vi "camera mjpeg.vi"(11 "CameraDevRef":T1) -> ()   [LabVIEW 2014]
uses:
  <vilib>/Rock Robotics/WPI/Camera/WPI_CameraDevRef.ctl
  <vilib>/Rock Robotics/WPI/Camera/WPI_CameraSettings Operations.ctl
  typedefs/vision/vision enable.ctl
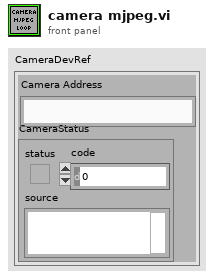
[diagram p1: front panel]
types:
  T1 = typedef "WPI_CameraDevRef.ctl" = cluster{"Camera Address":string, "CameraStatus":errorcluster}
  T2 = typedef "WPI_CameraSettings Operations.ctl" = enum16{"Udate FPS", "Update Compression", "Update Size", "Update White Balance", "Update Brightness", "Update Sharpness", "Update Exposure", "Update Exposure Value", "Update Color Level", "Update Exp Priority", "Update Color Enable", "Update JPG", "Update MJPG", "Read and Clear", "Read", "Init"}
  T3 = typedef "vision enable.ctl" = enum16{"Enable", "Disable", "Stop"}
  T4 = typedef "WPI_CameraSettings Control.ctl" = cluster{"FPS":i32, "Compression":i32, "Size":i32, "White Balance":i32, "Brightness":i32, "Sharpness":i32, "Exposure":i32, "Color Level":i32, "Exposure Priority":i32, "Color Enable":i32, "JPG Loop":i32, "MJPG Loop":i32, "Exposure Value":i32}
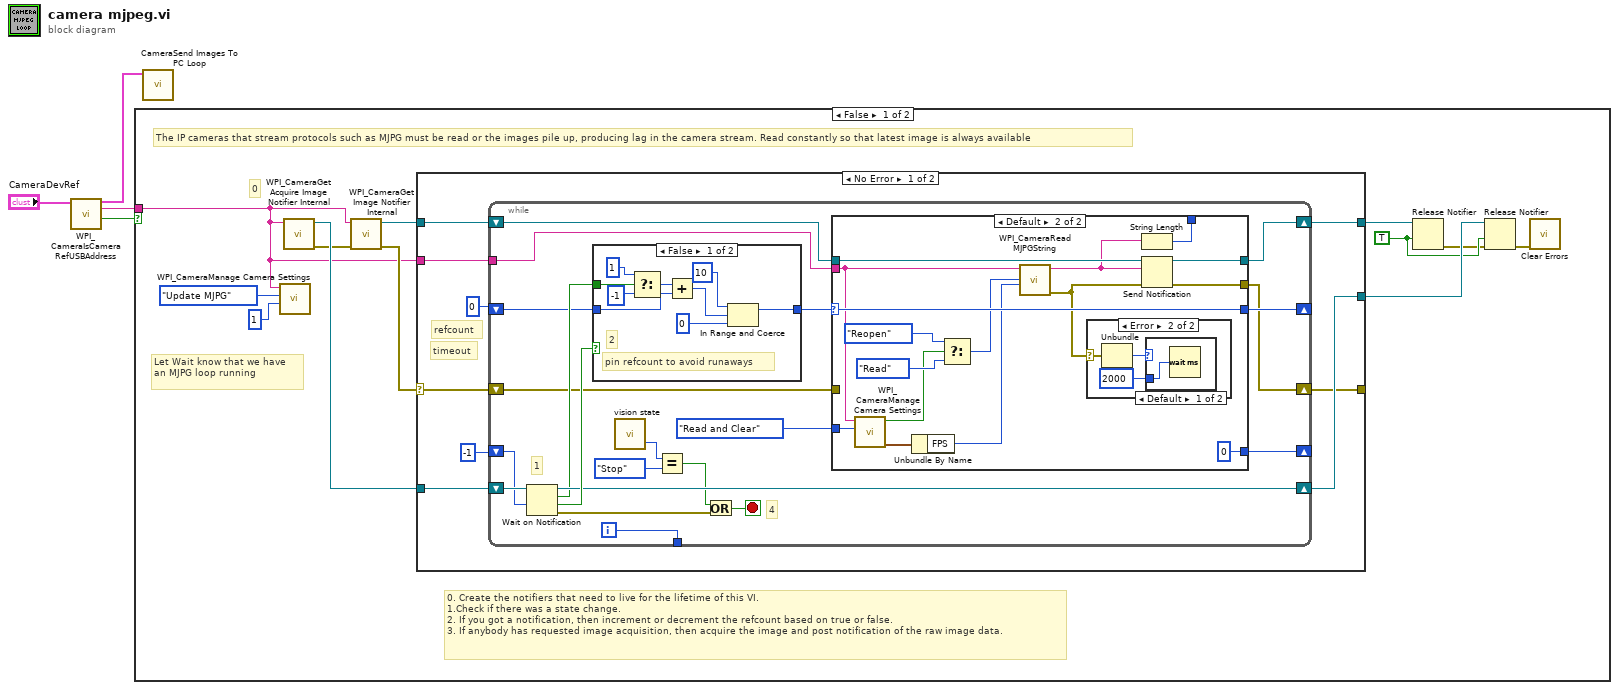
[diagram p0: block diagram]
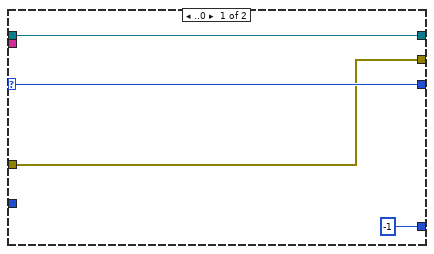
[diagram p2: hidden frame]
diagram:
  n1 = call <vilib>:"WPI_CameraIsCameraRefUSBAddress.vi"("CameraDevRef"="CameraDevRef") -> ("USB?"=w3:bool, "Camera Address Out"=w2:string, "CameraDevRef out"=w1:T1)  [unwired: 7 in, 1 out]
  n2 = case shown="False" w3 {
    tunnel: w2 -> [w6 _]
    frame False {
      w13 = TRUE ("force destroy? (F)")
      # "The IP cameras that stream protocols such as MJPG must be read or the images pile up, producing lag in the camera stream. Read constantly so that latest image is always available"
      # "0. Create the notifiers that need to live for the lifetime of this VI. \n1.Check if there was a state change.\n2. If you got a notification, then increment or decrement the refcount based on true or false.\n3. If anybody has requested image acquisition, then acquire the image and post notification of the raw image data."
      # "Let Wait know that we have\nan MJPG loop running"
      # "0"
      n3 = call <vilib>:"WPI_CameraManage Camera Settings.vi"("Value"=1, "Operation"=WPI_CameraSettings_Operations."Update MJPG", "Camera IP"=w6) -> ()  [unwired: 7 in, 2 out]
      n4 = call <vilib>:"WPI_CameraGet Acquire Image Notifier Internal.vi"("Camera Address"=w6) -> ("error out"=w10:errorcluster, "Acquire Image Notifier"=w11:refnum<notifier>)  [unwired: 1 in, 8 out]
      n5 = call <vilib>:"WPI_CameraGet Image Notifier Internal.vi"("error in (no error)"=w10, "Camera Address"=w6) -> ("error out"=w12:errorcluster, "Image Notifier"=w14:refnum<notifier>)  [unwired: 8 out]
      n6 = case shown="No Error" w12 {
        selector: w12 -> [w18 w83]
        tunnel: w6 -> [w25 _]
        tunnel: w11 -> [w24 w81]
        tunnel: w14 -> [w22 w82]
        tunnel: [w20 w82] -> w16
        tunnel: [w19 w81] -> w15
        tunnel: [w17 w83] -> _
        frame No Error {
          # "timeout"
          # "refcount"
          n7 = while {
            shift-right: [w44] -> w19
            shift-left: w24 -> [w46]
            tunnel: w25 -> [w41]
            shift-right: [w34] -> _
            shift-left: 0 -> [w42]
            shift-right: [w39] -> w20
            shift-left: w22 -> [w40]
            shift-right: [w37] -> _
            shift-left: -1 -> [w38]
            shift-right: [w33] -> w17
            shift-left: w18 -> [w36]
            tunnel: [w31] -> _
            i -> [w31]
            stop <- w28 stop-if-true
            # "4"
            # "1"
            n8 = Wait on Notification(notifier=w46, timeout in ms (-1)=w38) -> (notifier out=w44:refnum<notifier>, notification=w43:bool, timed out?=w45:bool, error out=w27:errorcluster)  [unwired: 1 in, 1 out]
            n9 = case shown="False" w45 {
              tunnel: w43 -> [w79 _]
              tunnel: w42 -> [w75 w80]
              tunnel: [w71 w80] -> w35
              frame False {
                # "pin refcount to avoid runaways"
                # "2"
                n10 = Select(t=1, s=w79, f=-1) -> (s? t:f=w76:i32)
                n11 = Add(x=w76, y=w75) -> (x+y=w72:i32)
                n12 = In Range and Coerce(upper limit=10, x=w72, lower limit=0) -> (coerced(x)=w71:i32)  [unwired: 1 out]
              }
              frame True {
              }
            }
            n13 = call "vision state.vi"() -> ("State Out"=w30:T3)  [unwired: 2 in, 1 out]
            n14 = Equal?(x=w30, y=vision_enable."Stop") -> (x = y?=w26:bool)
            n15 = Or(x=w26, y=w27) -> (x .or. y?=w28:bool)
            n16 = case shown="Default" w35 {
              selector: w35 -> [w49 w63]
              tunnel: w41 -> [_ w51]
              tunnel: w40 -> [w50 w66]
              tunnel: [w50 w65] -> w39
              tunnel: [-1 0] -> w37
              tunnel: w36 -> [w47 _]
              tunnel: [w49 w63] -> w34
              tunnel: [w47 w62] -> w33
              tunnel: [_ w56] -> _
              tunnel: WPI_CameraSettings_Operations."Read and Clear" ("Operation") -> [_ w52]
              frame ..0 {
              }
              frame Default {
                n17 = call <vilib>:"WPI_CameraManage Camera Settings.vi"("Operation"=w52, "Camera IP"=w51) -> ("Values"=w54:T4, "Changed"=w55:bool)  [unwired: 8 in]
                n18 = Unbundle By Name(w54) -> ("FPS"=w53:i32)
                n19 = Select(t=enum16{"Read", "Reopen", "Close"}."Reopen" ("Operation"), s=w55, f=enum16{"Read", "Reopen", "Close"}."Read" ("Operation")) -> (s? t:f=w58:enum16{"Read", "Reopen", "Close"})
                n20 = call <vilib>:"WPI_CameraRead MJPGString.vi"("fps"=w53, "Operation"=w58, "address"=w51) -> ("error out"=w61:errorcluster, "Raw Image Data"=w57:string)  [unwired: 7 in]
                n21 = case shown="Error" w61 {
                  selector: w61 -> [_ w69]
                  frame No Error {
                  }
                  frame Error {
                    n22 = Unbundle(w69) -> ("code"=w68:i32)  [unwired: 2 out]
                    n23 = case shown="Default" w68 {
                      tunnel: u32 2000 ("milliseconds to wait") -> [w70 _]
                      frame Default {
                        n24 = Wait (ms)(milliseconds to wait=w70) -> ()  [unwired: 1 out]
                      }
                      frame 56 {
                      }
                    }
                  }
                }
                n25 = String Length(string=w57) -> (length=w56:i32)
                n26 = Send Notification(notification=w57, notifier=w66, error in (no error)=w61) -> (notifier out=w65:refnum<notifier>, error out=w62:errorcluster)
              }
            }
          }
        }
        frame Error {
        }
      }
      n27 = Release Notifier(notifier=w16, force destroy? (F)=w13) -> (error out=w9:errorcluster)  [unwired: 1 in, 2 out]
      n28 = Release Notifier(notifier=w15, force destroy? (F)=w13, error in (no error)=w9) -> (error out=w5:errorcluster)  [unwired: 2 out]
      n29 = call <vilib>:"Clear Errors.vi"("error in (no error)"=w5) -> ()  [unwired: 1 in, 6 out]
    }
    frame True {
      # "The USB cameras may need to be forwarded over ethernet. Read, compress, and send to the Dashbd."
    }
  }
  n30 = call "CameraSend Images To PC Loop.vi"("CameraDevRef"=w1) -> ()  [unwired: 11 in]
